vi "Autonomous Independent.vi"   [LabVIEW 2013]
doc: "This VI is called when autonomous begins, and will automatically be terminated when autonomous ends. You can carry out timed or sensor driven robot movement independently without needing to return to the caller."
uses:
  Robot Global Data.vi
  <vilib>/Rock Robotics/WPI/Joystick/WPI_JoystickGetSetRefNum.vi
panel:
  # "Be sure to right-click and choose Data Operations>>Make Current Value default if you want to save the array values with the VI"
types:
  T1 = typedef "WPI_JoystickDevRef.ctl" = cluster{"Device":T2}
  T2 = typedef "WPI_JoystickDeviceEnum.ctl" = enum16{"USB 1", "USB 2", "USB 3", "USB 4", "Kinect 1", "Kinect 2"}
  T3 = cluster{"axis 1 (x)":dbl, "axis 2 (y)":dbl, "axis 3 (throttle)":dbl, "axis 4":dbl, "axis 5":dbl, "axis 6":dbl}
  T4 = typedef "WPI_MotorControlDeviceRef.ctl" = cluster{"DeviceStatus":errorcluster, "Type":enum16{"PWM", "CAN"}, "PWM":cluster{"Digital Module":T5, "PWM Channel":T6, "DeadBand":T7}, "CAN":cluster{"Device Number":u8, "Control Mode":T8, "Semaphore":T9, "Max Vout":dbl}, "Invert":bool, "TransformRef":T10, "InvTransformRef":T10}
  T5 = typedef "FPGA_TypedefDigitalModule.ctl" = enum16{"Digital Module 1", "Digital Module 2"}
  T6 = typedef "FPGA_DIOPWMChannel.ctl" = enum8{"PWM 1", "PWM 2", "PWM 3", "PWM 4", "PWM 5", "PWM 6", "PWM 7", "PWM 8", "PWM 9", "PWM 10", "Invalid"}
  T7 = typedef "WPI_PWMDeadband.ctl" = cluster{"Name":string, "maxPositivePwm":i32, "minPositivePwm":i32, "centerPwm":i32, "maxNegativePwm":i32, "minNegativePwm":i32, "angularRange":u16}
  T8 = typedef "WPI_CANJaguar_ControlMode.ctl" = enum8{"Percent VBus", "Current", "Speed", "Position", "Voltage"}
  T9 = typedef "Semaphore RefNum" = refnum<k1>
  T10 = typedef "WPI_PWMTransform_ConPane.ctl" = refnum<vi>
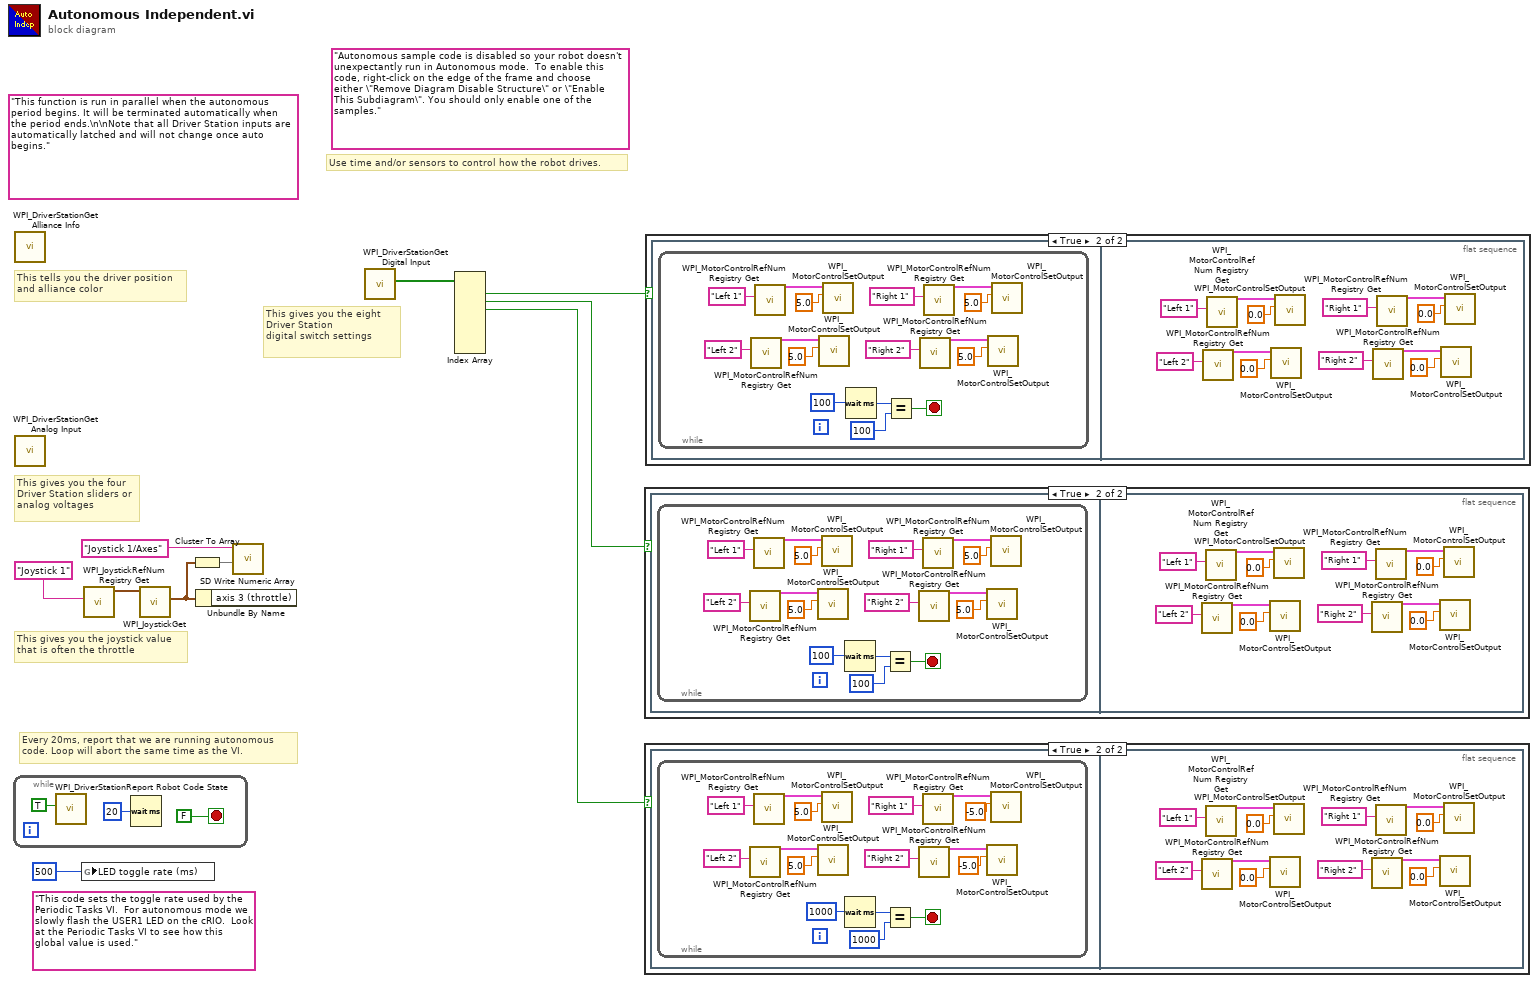
[diagram p0: block diagram]
diagram:
  (unwired) "This code sets the toggle rate used by the Periodic Tasks VI.  For autonomous mode we slowly flash the USER1 LED on the cRIO.  Look at the Periodic Tasks VI to see how this global value is used."
  (unwired) "Autonomous sample code is disabled so your robot doesn't unexpectantly run in Autonomous mode.  To enable this code, right-click on the edge of the frame and choose either \"Remove Diagram Disable Structure\" or \"Enable This Subdiagram\". You should only enable one of the samples."
  (unwired) "This function is run in parallel when the autonomous period begins. It will be terminated automatically when the period ends.\n\nNote that all Driver Station inputs are automatically latched and will not change once auto begins."
  # "Every 20ms, report that we are running autonomous\ncode. Loop will abort the same time as the VI."
  # "This gives you the joystick value\nthat is often the throttle"
  # "Use time and/or sensors to control how the robot drives."
  # "This tells you the driver position\nand alliance color"
  # "This gives you the eight Driver Station\ndigital switch settings"
  # "This gives you the four\nDriver Station sliders or\nanalog voltages"
  n1 = while {
    stop <- FALSE stop-if-true
    n2 = call <vilib>:"WPI_DriverStationReport Robot Code State.vi"("Autonomous"=TRUE) -> ()  [unwired: 10 in, 1 out]
    n3 = Wait (ms)(milliseconds to wait=u32 20) -> ()  [unwired: 1 out]
  }
  n4 = call <vilib>:"WPI_DriverStationGet Alliance Info.vi"() -> ()  [unwired: 12 out]
  n5 = call <vilib>:"WPI_DriverStationGet Analog Input.vi"() -> ()  [unwired: 12 out]
  n6 = global write "Robot Global Data.vi" "LED toggle rate (ms)"(u32 500 ("LED ms toggle rate")) -> ()
  n7 = call <vilib>:"WPI_JoystickRefNum Registry Get.vi"("refnum name"="Joystick 1") -> ("JoystickDevRef"=w9:T1)  [unwired: 1 in, 9 out]
  n8 = call <vilib>:"WPI_JoystickGet.vi"("JoystickDevRef"=w9) -> ("Axes"=w6:T3)  [unwired: 1 in, 5 out]
  n9 = Cluster To Array(cluster=w6) -> (array=w7:dbl[])
  n10 = Unbundle By Name(w6) -> ()  [unwired: 1 out]
  n11 = call <vilib>:"SD Write Numeric Array.vi"("Numeric Array"=w7, "Name"="Joystick 1/Axes") -> ()  [unwired: 8 in, 2 out]
  n12 = call <vilib>:"WPI_DriverStationGet Digital Input.vi"() -> ("Driver Station Digital Input (1-8)"=w4:bool[])  [unwired: 11 out]
  n13 = Index Array(array=w4) -> (element #1=w3:bool, element #2=w2:bool, element #3=w1:bool)  [unwired: 8 in, 5 out]
  n14 = case shown="True" w2 {
    frame False {
    }
    frame True {
      n15 = flat-sequence {
        frame #0 {
          n16 = while {
            stop <- w14 stop-if-true
            n17 = call <vilib>:"WPI_MotorControlRefNum Registry Get.vi"("refnum name"="Left 2") -> ("MotorControlDevRef"=w20:T4)  [unwired: 9 in, 1 out]
            n18 = call <vilib>:"WPI_MotorControlRefNum Registry Get.vi"("refnum name"="Left 1") -> ("MotorControlDevRef"=w22:T4)  [unwired: 9 in, 1 out]
            n19 = call <vilib>:"WPI_MotorControlSetOutput.vi"("Output"=5.0, "MotorControlDevRef"=w20) -> ()  [unwired: 7 in, 3 out]
            n20 = call <vilib>:"WPI_MotorControlSetOutput.vi"("Output"=5.0, "MotorControlDevRef"=w22) -> ()  [unwired: 7 in, 3 out]
            n21 = Wait (ms)(milliseconds to wait=100) -> (millisecond timer value=w16:u32)
            n22 = Equal?(x=w16, y=100) -> (x = y?=w14:bool)
            n23 = call <vilib>:"WPI_MotorControlRefNum Registry Get.vi"("refnum name"="Right 2") -> ("MotorControlDevRef"=w26:T4)  [unwired: 9 in, 1 out]
            n24 = call <vilib>:"WPI_MotorControlRefNum Registry Get.vi"("refnum name"="Right 1") -> ("MotorControlDevRef"=w28:T4)  [unwired: 9 in, 1 out]
            n25 = call <vilib>:"WPI_MotorControlSetOutput.vi"("Output"=5.0, "MotorControlDevRef"=w26) -> ()  [unwired: 7 in, 3 out]
            n26 = call <vilib>:"WPI_MotorControlSetOutput.vi"("Output"=5.0, "MotorControlDevRef"=w28) -> ()  [unwired: 7 in, 3 out]
          }
        }
        frame #1 {
          n27 = call <vilib>:"WPI_MotorControlRefNum Registry Get.vi"("refnum name"="Left 2") -> ("MotorControlDevRef"=w32:T4)  [unwired: 9 in, 1 out]
          n28 = call <vilib>:"WPI_MotorControlRefNum Registry Get.vi"("refnum name"="Left 1") -> ("MotorControlDevRef"=w34:T4)  [unwired: 9 in, 1 out]
          n29 = call <vilib>:"WPI_MotorControlSetOutput.vi"("Output"=0.0, "MotorControlDevRef"=w32) -> ()  [unwired: 7 in, 3 out]
          n30 = call <vilib>:"WPI_MotorControlSetOutput.vi"("Output"=0.0, "MotorControlDevRef"=w34) -> ()  [unwired: 7 in, 3 out]
          n31 = call <vilib>:"WPI_MotorControlRefNum Registry Get.vi"("refnum name"="Right 2") -> ("MotorControlDevRef"=w38:T4)  [unwired: 9 in, 1 out]
          n32 = call <vilib>:"WPI_MotorControlRefNum Registry Get.vi"("refnum name"="Right 1") -> ("MotorControlDevRef"=w40:T4)  [unwired: 9 in, 1 out]
          n33 = call <vilib>:"WPI_MotorControlSetOutput.vi"("Output"=0.0, "MotorControlDevRef"=w38) -> ()  [unwired: 7 in, 3 out]
          n34 = call <vilib>:"WPI_MotorControlSetOutput.vi"("Output"=0.0, "MotorControlDevRef"=w40) -> ()  [unwired: 7 in, 3 out]
        }
      }
    }
  }
  n35 = case shown="True" w1 {
    frame False {
    }
    frame True {
      n36 = flat-sequence {
        frame #0 {
          n37 = while {
            stop <- w42 stop-if-true
            n38 = call <vilib>:"WPI_MotorControlRefNum Registry Get.vi"("refnum name"="Left 2") -> ("MotorControlDevRef"=w48:T4)  [unwired: 9 in, 1 out]
            n39 = call <vilib>:"WPI_MotorControlRefNum Registry Get.vi"("refnum name"="Left 1") -> ("MotorControlDevRef"=w50:T4)  [unwired: 9 in, 1 out]
            n40 = call <vilib>:"WPI_MotorControlSetOutput.vi"("Output"=5.0, "MotorControlDevRef"=w48) -> ()  [unwired: 7 in, 3 out]
            n41 = call <vilib>:"WPI_MotorControlSetOutput.vi"("Output"=5.0, "MotorControlDevRef"=w50) -> ()  [unwired: 7 in, 3 out]
            n42 = Wait (ms)(milliseconds to wait=1000) -> (millisecond timer value=w44:u32)
            n43 = Equal?(x=w44, y=1000) -> (x = y?=w42:bool)
            n44 = call <vilib>:"WPI_MotorControlRefNum Registry Get.vi"("refnum name"="Right 2") -> ("MotorControlDevRef"=w54:T4)  [unwired: 9 in, 1 out]
            n45 = call <vilib>:"WPI_MotorControlRefNum Registry Get.vi"("refnum name"="Right 1") -> ("MotorControlDevRef"=w56:T4)  [unwired: 9 in, 1 out]
            n46 = call <vilib>:"WPI_MotorControlSetOutput.vi"("Output"=-5.0, "MotorControlDevRef"=w54) -> ()  [unwired: 7 in, 3 out]
            n47 = call <vilib>:"WPI_MotorControlSetOutput.vi"("Output"=-5.0, "MotorControlDevRef"=w56) -> ()  [unwired: 7 in, 3 out]
          }
        }
        frame #1 {
          n48 = call <vilib>:"WPI_MotorControlRefNum Registry Get.vi"("refnum name"="Left 2") -> ("MotorControlDevRef"=w60:T4)  [unwired: 9 in, 1 out]
          n49 = call <vilib>:"WPI_MotorControlRefNum Registry Get.vi"("refnum name"="Left 1") -> ("MotorControlDevRef"=w62:T4)  [unwired: 9 in, 1 out]
          n50 = call <vilib>:"WPI_MotorControlSetOutput.vi"("Output"=0.0, "MotorControlDevRef"=w60) -> ()  [unwired: 7 in, 3 out]
          n51 = call <vilib>:"WPI_MotorControlSetOutput.vi"("Output"=0.0, "MotorControlDevRef"=w62) -> ()  [unwired: 7 in, 3 out]
          n52 = call <vilib>:"WPI_MotorControlRefNum Registry Get.vi"("refnum name"="Right 2") -> ("MotorControlDevRef"=w66:T4)  [unwired: 9 in, 1 out]
          n53 = call <vilib>:"WPI_MotorControlRefNum Registry Get.vi"("refnum name"="Right 1") -> ("MotorControlDevRef"=w68:T4)  [unwired: 9 in, 1 out]
          n54 = call <vilib>:"WPI_MotorControlSetOutput.vi"("Output"=0.0, "MotorControlDevRef"=w66) -> ()  [unwired: 7 in, 3 out]
          n55 = call <vilib>:"WPI_MotorControlSetOutput.vi"("Output"=0.0, "MotorControlDevRef"=w68) -> ()  [unwired: 7 in, 3 out]
        }
      }
    }
  }
  n56 = case shown="True" w3 {
    frame False {
    }
    frame True {
      n57 = flat-sequence {
        frame #0 {
          n58 = while {
            stop <- w70 stop-if-true
            n59 = call <vilib>:"WPI_MotorControlRefNum Registry Get.vi"("refnum name"="Left 2") -> ("MotorControlDevRef"=w76:T4)  [unwired: 9 in, 1 out]
            n60 = call <vilib>:"WPI_MotorControlRefNum Registry Get.vi"("refnum name"="Left 1") -> ("MotorControlDevRef"=w78:T4)  [unwired: 9 in, 1 out]
            n61 = call <vilib>:"WPI_MotorControlSetOutput.vi"("Output"=5.0, "MotorControlDevRef"=w76) -> ()  [unwired: 7 in, 3 out]
            n62 = call <vilib>:"WPI_MotorControlSetOutput.vi"("Output"=5.0, "MotorControlDevRef"=w78) -> ()  [unwired: 7 in, 3 out]
            n63 = Wait (ms)(milliseconds to wait=100) -> (millisecond timer value=w72:u32)
            n64 = Equal?(x=w72, y=100) -> (x = y?=w70:bool)
            n65 = call <vilib>:"WPI_MotorControlRefNum Registry Get.vi"("refnum name"="Right 2") -> ("MotorControlDevRef"=w82:T4)  [unwired: 9 in, 1 out]
            n66 = call <vilib>:"WPI_MotorControlRefNum Registry Get.vi"("refnum name"="Right 1") -> ("MotorControlDevRef"=w84:T4)  [unwired: 9 in, 1 out]
            n67 = call <vilib>:"WPI_MotorControlSetOutput.vi"("Output"=5.0, "MotorControlDevRef"=w82) -> ()  [unwired: 7 in, 3 out]
            n68 = call <vilib>:"WPI_MotorControlSetOutput.vi"("Output"=5.0, "MotorControlDevRef"=w84) -> ()  [unwired: 7 in, 3 out]
          }
        }
        frame #1 {
          n69 = call <vilib>:"WPI_MotorControlRefNum Registry Get.vi"("refnum name"="Left 2") -> ("MotorControlDevRef"=w88:T4)  [unwired: 9 in, 1 out]
          n70 = call <vilib>:"WPI_MotorControlRefNum Registry Get.vi"("refnum name"="Left 1") -> ("MotorControlDevRef"=w90:T4)  [unwired: 9 in, 1 out]
          n71 = call <vilib>:"WPI_MotorControlSetOutput.vi"("Output"=0.0, "MotorControlDevRef"=w88) -> ()  [unwired: 7 in, 3 out]
          n72 = call <vilib>:"WPI_MotorControlSetOutput.vi"("Output"=0.0, "MotorControlDevRef"=w90) -> ()  [unwired: 7 in, 3 out]
          n73 = call <vilib>:"WPI_MotorControlRefNum Registry Get.vi"("refnum name"="Right 2") -> ("MotorControlDevRef"=w94:T4)  [unwired: 9 in, 1 out]
          n74 = call <vilib>:"WPI_MotorControlRefNum Registry Get.vi"("refnum name"="Right 1") -> ("MotorControlDevRef"=w96:T4)  [unwired: 9 in, 1 out]
          n75 = call <vilib>:"WPI_MotorControlSetOutput.vi"("Output"=0.0, "MotorControlDevRef"=w94) -> ()  [unwired: 7 in, 3 out]
          n76 = call <vilib>:"WPI_MotorControlSetOutput.vi"("Output"=0.0, "MotorControlDevRef"=w96) -> ()  [unwired: 7 in, 3 out]
        }
      }
    }
  }
